vi "HEWH Calibrate Totalized Gallons.vi"(10 "Calibration Coefficients":T1, 11 "Gallon Input":dbl) -> (3 "AdjGal Output":dbl)   [LabVIEW 2014]
uses:
  Type Definitions/HEWH Calibration Coefficients.ctl
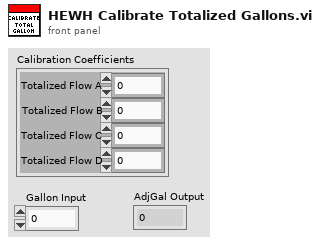
[diagram p1: front panel]
types:
  T1 = typedef "HEWH Calibration Coefficients.ctl" = cluster{"Totalized Flow A":dbl, "Totalized Flow B":dbl, "Totalized Flow C":dbl, "Totalized Flow D":dbl}
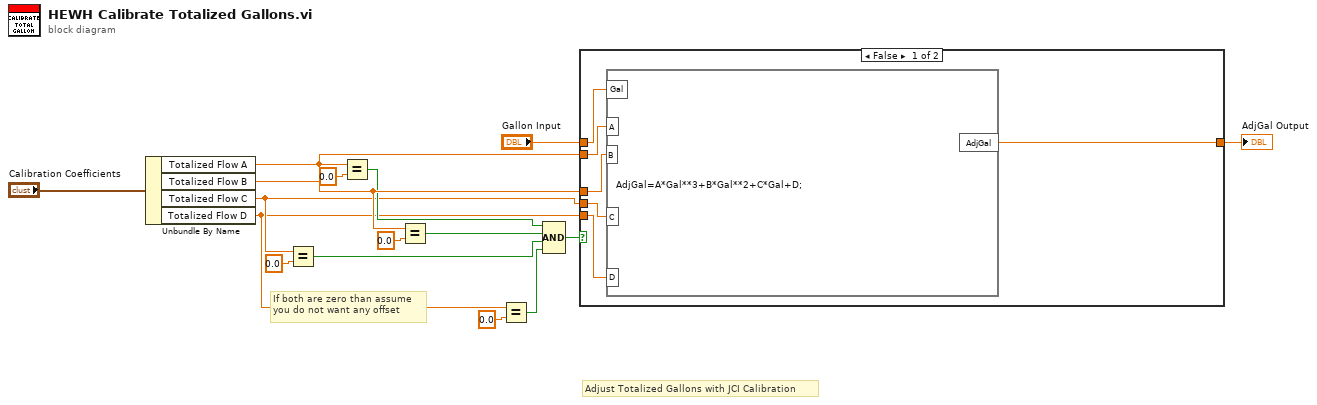
[diagram p0: block diagram]
diagram:
  # "If both are zero than assume \nyou do not want any offset"
  # "Adjust Totalized Gallons with JCI Calibration"
  n1 = Unbundle By Name("Calibration Coefficients") -> ("Totalized Flow A"=w15:dbl, "Totalized Flow B"=w16:dbl, "Totalized Flow C"=w2:dbl, "Totalized Flow D"=w1:dbl)
  n2 = Equal?(x=w2, y=0.0) -> (x = y?=w4:bool)
  n3 = Equal?(x=w15, y=0.0) -> (x = y?=w10:bool)
  n4 = Equal?(x=w16, y=0.0) -> (x = y?=w11:bool)
  n5 = Equal?(x=w1, y=0.0) -> (x = y?=w3:bool)
  n6 = Compound Arithmetic op=AND(w10, w11, w4, w3) -> (w12:bool)
  n7 = case shown="False" w12 {
    tunnel: "Gallon Input" -> [w21 w23]
    tunnel: [w22 w23] -> w14
    tunnel: w15 -> [w20 _]
    tunnel: w16 -> [w19 _]
    tunnel: w2 -> [w18 _]
    tunnel: w1 -> [w17 _]
    frame False {
      n8 = formula code="AdjGal=A*Gal**3+B*Gal**2+C*Gal+D;"("Gal"=w21, "A"=w20, "B"=w19, "C"=w18, "D"=w17) -> ("AdjGal"=w22:dbl)
    }
    frame True {
    }
  }
  "AdjGal Output" <- w14
